vi "Set Sessions_Controller_Screen.vi"(11 "Semiconductor Module Context":T1) -> (0 "error out":errorcluster)   [LabVIEW 2013]
uses:
  <vilib>/NI_TestStand_SemiconductorModule/NI_TestStand_Semiconductor_Module.lvlibp/PinMap/General/SemiconductorModuleContext.ctl
  <vilib>/NI_TestStand_SemiconductorModule/NI_TestStand_Semiconductor_Module.lvlibp
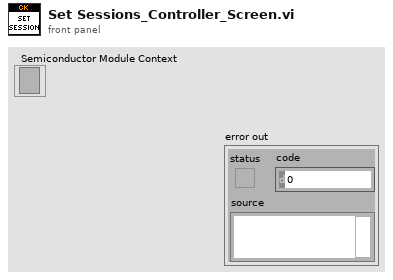
[diagram p1: front panel]
types:
  T1 = typedef "NI_TestStand_Semiconductor_Module.lvlibp/SemiconductorModuleContext.ctl" = refnum<k7>
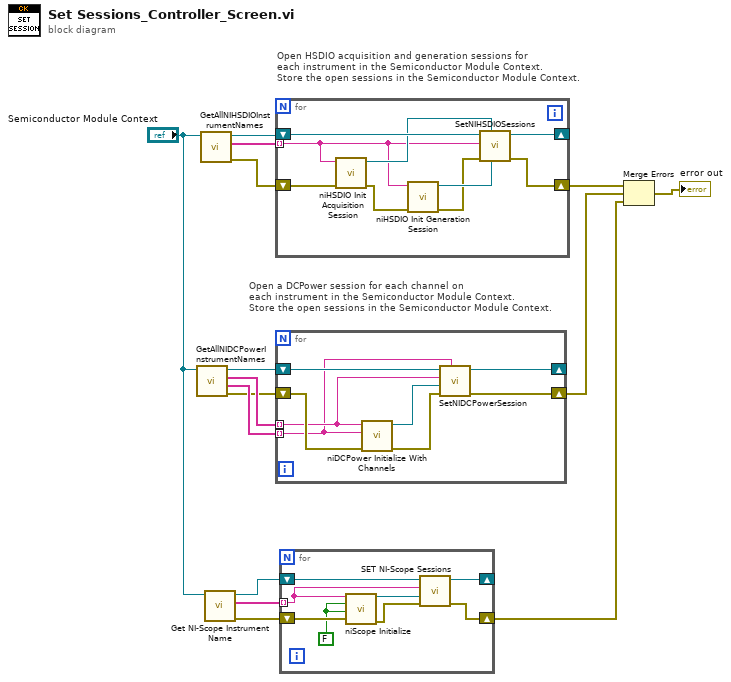
[diagram p0: block diagram]
diagram:
  # "Open a DCPower session for each channel on \neach instrument in the Semiconductor Module Context.\nStore the open sessions in the Semiconductor Module Context."
  # "Open HSDIO acquisition and generation sessions for\neach instrument in the Semiconductor Module Context.\nStore the open sessions in the Semiconductor Module Context."
  n1 = call <vilib>:"GetAllNIDCPowerInstrumentNames.vi"("Semiconductor Module Context"="Semiconductor Module Context") -> ("error out"=w8:errorcluster, "Channel Ids"=w9:string[], "Instrument Names"=w14:string[], "Semiconductor Module Context Out"=w13:T1)  [unwired: 7 in]
  n2 = call <vilib>:"GetAllNIHSDIOInstrumentNames.vi"("Semiconductor Module Context"="Semiconductor Module Context") -> ("error out"=w6:errorcluster, "Instrument Names"=w15:string[], "Semiconductor Module Context Out"=w7:T1)  [unwired: 8 in]
  n3 = call "Get NI-Scope Instrument Name.vi"("Semiconductor Module Context"="Semiconductor Module Context") -> ("Error Out"=w5:errorcluster, "Instrument Names"=w3:string[], "Semiconductor Module Context Out"=w4:T1)  [unwired: 7 in, 1 out]
  n4 = for {
    tunnel: w15 -> [w17] mode=indexing
    shift-right: [w19] -> w12
    shift-left: w6 -> [w24]
    shift-right: [w21] -> _
    shift-left: w7 -> [w23]
    n5 = call <instrlib>:"niHSDIO Init Acquisition Session.vi"("error in (no error)"=w24, "resource name"=w17) -> ("error out"=w18:errorcluster, "instrument handle out"=w22:refnum<k15>)  [unwired: 8 in]
    n6 = call <instrlib>:"niHSDIO Init Generation Session.vi"("error in (no error)"=w18, "resource name"=w17) -> ("error out"=w16:errorcluster, "instrument handle out"=w20:refnum<k15>)  [unwired: 8 in]
    n7 = call <vilib>:"SetNIHSDIOSessions.vi"("Generation Session"=w20, "Acquisition Session"=w22, "error in (no error)"=w16, "Instrument Name"=w17, "Semiconductor Module Context"=w23) -> ("error out"=w19:errorcluster, "Semiconductor Module Context Out"=w21:T1)  [unwired: 5 in]
  }
  n8 = for {
    tunnel: w14 -> [w28] mode=indexing
    shift-right: [w31] -> _
    shift-left: w13 -> [w32]
    shift-right: [w30] -> w11
    shift-left: w8 -> [w29]
    tunnel: w9 -> [w25] mode=indexing
    n9 = call <instrlib>:"niDCPower Initialize With Channels.vi"("error in (no error)"=w29, "channels"=w25, "resource name"=w28) -> ("error out"=w27:errorcluster, "instrument handle out"=w26:refnum<k15>)  [unwired: 7 in]
    n10 = call <vilib>:"SetNIDCPowerSession.vi"("Channel Id"=w25, "error in (no error)"=w27, "Instrument Session"=w26, "Instrument Name"=w28, "Semiconductor Module Context"=w32) -> ("error out"=w30:errorcluster, "Semiconductor Module Context Out"=w31:T1)  [unwired: 5 in]
  }
  n11 = for {
    tunnel: w3 -> [w36] mode=indexing
    shift-right: [w33] -> _
    shift-left: w4 -> [w38]
    shift-right: [w34] -> w1
    shift-left: w5 -> [w40]
    w39 = FALSE ("reset device")
    n12 = call <instrlib>:"niScope Initialize.vi"("resource name"=w36, "id query"=w39, "reset device"=w39, "error in"=w40) -> ("instrument handle"=w37:refnum<k15>, "error out"=w35:errorcluster)  [unwired: 10 in]
    n13 = call "SET NI-Scope Sessions.vi"("error in (no error)"=w35, "Instrument Handle In"=w37, "Instrument Name"=w36, "Semiconductor Module Context"=w38) -> ("error out"=w34:errorcluster, "Semiconductor Module Context Out"=w33:T1)  [unwired: 6 in]
  }
  n14 = Merge Errors(w12, w11, w1) -> (→"error out":errorcluster)
